vi "Start Metric.vi"(7 "Metrics Reverse":T1, 8 "error in (no error)":errorcluster, 10 "Metric":string, 11 "Module in":refnum<class "Module.lvclass">) -> (0 "error out":errorcluster, 3 "Module out":refnum<class "Module.lvclass">, 5 "Forward":T2)   [LabVIEW 2020, in "Volatus.lvlib" / "Module.lvclass"]
uses:
  Module.lvclass
  Metrics Forward.ctl
  Metrics Reverse.ctl
  Module.lvclass/Module.ctl
  MessageQ/MessageQ.lvclass/MessageQ.ctl
  Forward Metric.vi
  Parent Q.vi
  MessageQ/Is Null.vi
  MessageQ/Send.vi
  <vilib>/ptbypt/NI_PtbyPt.lvlib
  Volatus.lvlib
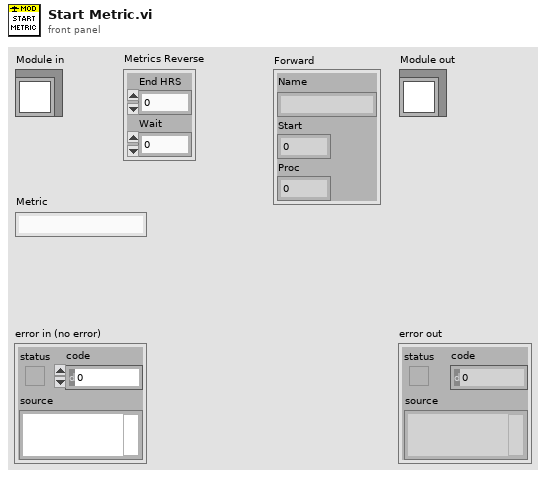
[diagram p1: front panel]
types:
  T1 = typedef "Volatus.lvlib/Metrics Reverse.ctl" = cluster{"End HRS":dbl, "Wait":dbl}
  T2 = typedef "Volatus.lvlib/Metrics Forward.ctl" = cluster{"Name":string, "Start":dbl, "Proc":dbl}
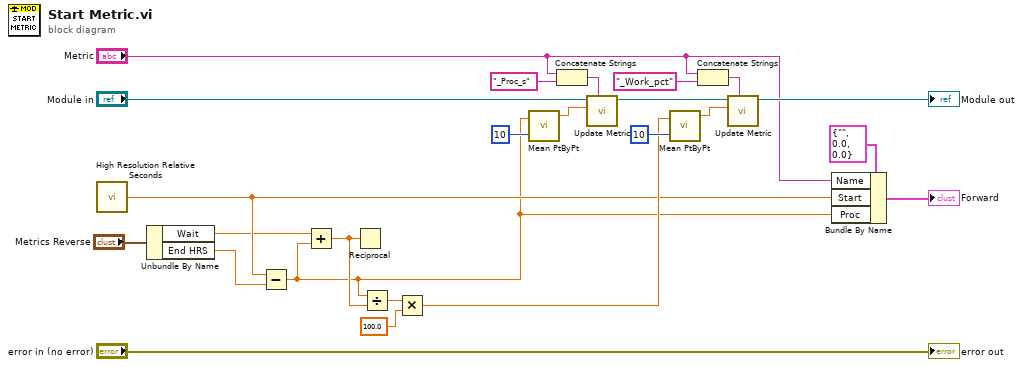
[diagram p0: block diagram]
diagram:
  n1 = call <vilib>:"High Resolution Relative Seconds.vi"() -> ("relative seconds"=w7:dbl)
  n2 = Unbundle By Name("Metrics Reverse") -> ("Wait"=w4:dbl, "End HRS"=w3:dbl)
  n3 = Subtract(x=w7, y=w3) -> (x-y=w2:dbl)
  n4 = Add(x=w4, y=w2) -> (x+y=w10:dbl)
  n5 = Reciprocal(x=w10) -> ()  [unwired: 1 out]
  n6 = Divide(x=w2, y=w10) -> (x/y=w15:dbl)
  n7 = Multiply(x=w15, y=100.0) -> (x*y=w11:dbl)
  n8 = call <vilib>:"Mean PtByPt.vi"("x"=w2, "sample length"=10) -> ("mean"=w20:dbl)  [unwired: 2 in, 1 out]
  n9 = Concatenate Strings("Metric", "_Proc_s" ("string")) -> (w22:string)
  n10 = call "Update Metric.vi"("Metric"=w22, "Value"=w20, "Module in"="Module in") -> ("Module out"=w13:refnum<class "Module.lvclass">)  [unwired: 7 in, 1 out]
  n11 = call <vilib>:"Mean PtByPt.vi"("x"=w11, "sample length"=10) -> ("mean"=w19:dbl)  [unwired: 2 in, 1 out]
  n12 = Concatenate Strings("Metric", "_Work_pct" ("string")) -> (w17:string)
  n13 = call "Update Metric.vi"("Metric"=w17, "Value"=w19, "Module in"=w13) -> ("Module out"=→"Module out":refnum<class "Module.lvclass">)  [unwired: 7 in, 1 out]
  n14 = Bundle By Name(cluster=T2 {"Name"="", "Start"=0.0, "Proc"=0.0} ("Metrics Forward"), "Name"="Metric", "Start"=w7, "Proc"=w2) -> (→"Forward":T2)
  "error out" <- "error in (no error)"
